vi "Add Scrollback Lines.vi"(8 "error in (no error)":errorcluster, 10 "Lines":refnum<class "TermLine.lvclass">[](array[class]), 11 "TermBuffer in":refnum<class "TermBuffer.lvclass">) -> (0 "error out":errorcluster, 3 "TermBuffer out":refnum<class "TermBuffer.lvclass">)   [LabVIEW 2020, in "Terminal.lvlib" / "TermBuffer.lvclass"]
uses:
  TermBuffer.lvclass
  TermBuffer.lvclass/TermBuffer.ctl
  TermLine/TermLine.lvclass
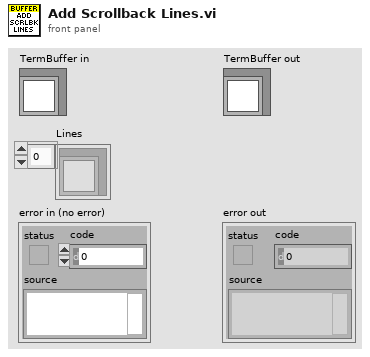
[diagram p1: front panel]
types:
  T1 = typedef "Terminal.lvlib/TermBuffer.lvclass/Ref Data.ctl" = cluster{"Lines":refnum<class "TermLine.lvclass">[]}
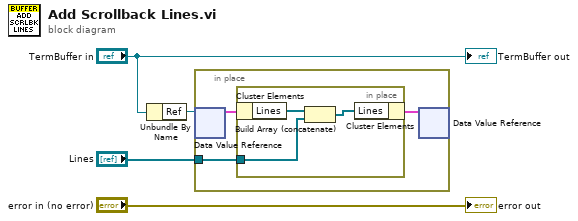
[diagram p0: block diagram]
diagram:
  n1 = Unbundle By Name("TermBuffer in") -> ("Ref"=w3:refnum<data-value>)
  n2 = in-place {
    in-place-border: "Lines" -> [w5]
    n3 = in-place-dvr #1(w3) -> (w7:T1)  [unwired: 1 out]
    n4 = in-place {
      in-place-border: w5 -> [w9]
      n5 = in-place-cluster #2(w7) -> ("Lines"=w10:refnum<class "TermLine.lvclass">[])
      n6 = Build Array (concatenate)(w10, w9) -> (w8:refnum<class "TermLine.lvclass">[])
      n7 = in-place-cluster #2("Lines"=w8) -> (w6:T1)
    }
    n8 = in-place-dvr #1(w6) -> ()  [unwired: 2 out]
  }
  "error out" <- "error in (no error)"
  "TermBuffer out" <- "TermBuffer in"
